vi "SPO2.vi"(5 "A":dbl=110.0 format="%#_13g", 7 "B":dbl=25.0 format="%#_13g", 8 "Inicial":u32, 9 "AMB":i16, 10 "IR":i16, 11 "RED":i16) -> (1 "Inicial Time Out":u32, 2 "Valor Medio":string, 3 "SpO2":string)   [LabVIEW 2013]
uses:
  <vilib>/Analysis/baseanly.llb/Mean (DBL).vi
  <vilib>/Analysis/NI_AALBase.lvlib
panel:
  out "Spo2 Array":dbl[](array[numeric])
  out "R":dbl
  out "VrmsIR":dbl
  out "VrmsRed":dbl
  out "VppIR":i16
  out "VppRed":i16
  out "MIN IR":dbl
  out "MIN IR":dbl
  out "MAX  IR":dbl
  out "MAX RED":dbl
  out "RED_ARRAY":i32[](array[numeric])
  out "IR_ARRAY":i32[](array[numeric])
  out "AMB_ARRAY":i32[](array[numeric])
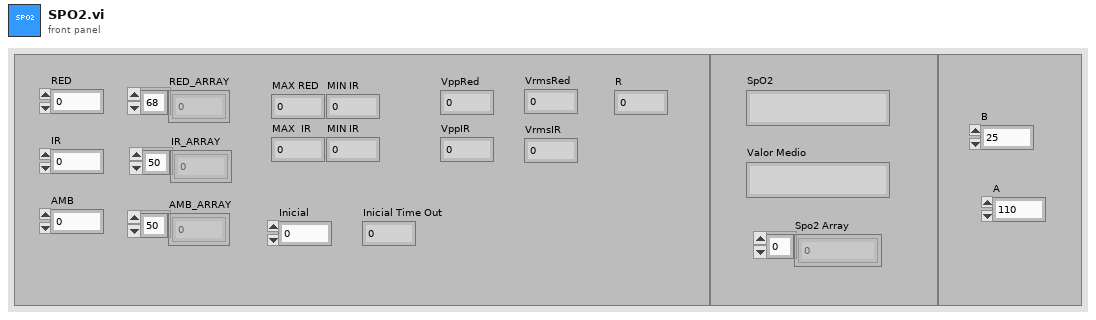
[diagram p1: front panel]
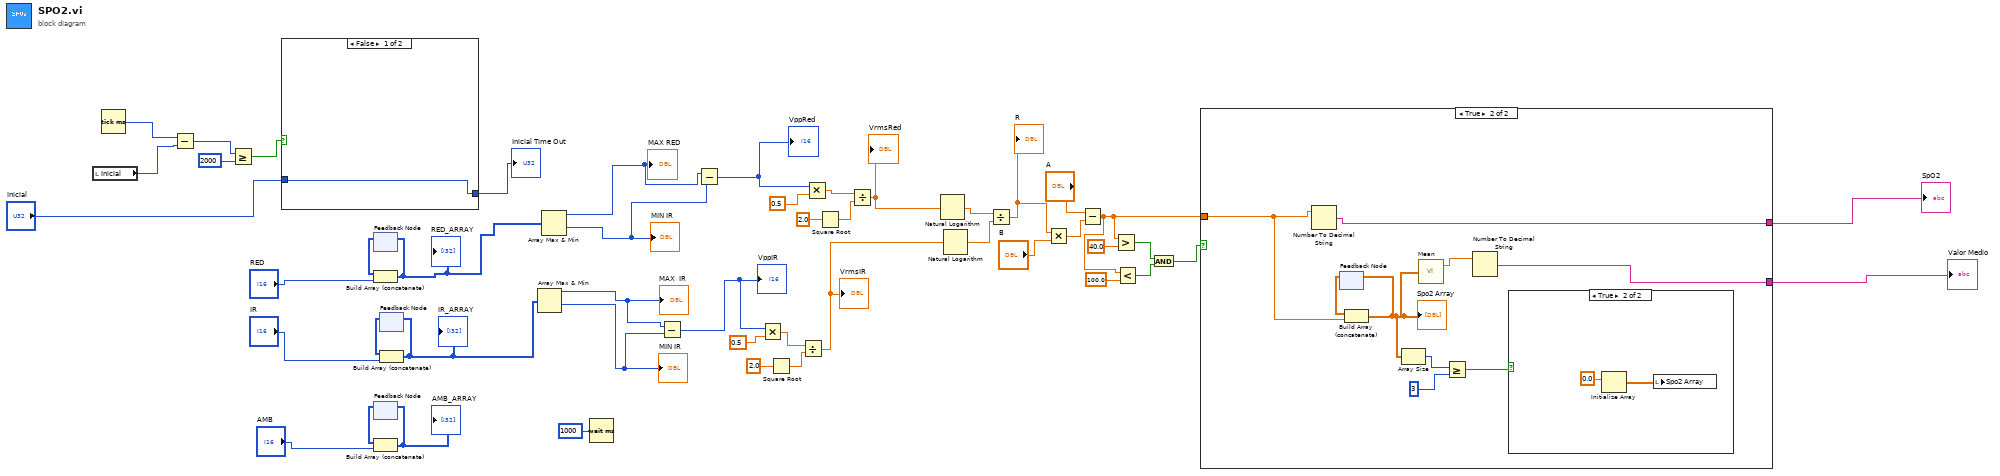
[diagram p0: block diagram]
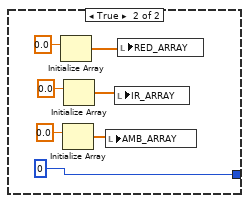
[diagram p2: hidden frame]
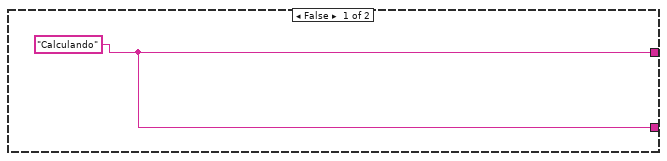
[diagram p3: hidden frame]
diagram:
  n1 = local read "Inicial"() -> (w3:u32)
  n2 = Tick Count (ms)() -> (millisecond timer value=w6:u32)
  n3 = Subtract(x=w6, y=w3) -> (x-y=w5:u32)
  n4 = Greater Or Equal?(x=w5, y=u32 2000) -> (x >= y?=w7:bool)
  n5 = case shown="False" w7 {
    tunnel: [w48 u32 0 ("Inicial Time")] -> w2
    tunnel: "Inicial" -> [w48 _]
    frame False {
    }
    frame True {
      n6 = Initialize Array(0.0 ("element")) -> (w52:dbl[])  [unwired: 1 in]
      n7 = Initialize Array(0.0 ("element")) -> (w50:dbl[])  [unwired: 1 in]
      n8 = Initialize Array(0.0 ("element")) -> (w51:dbl[])  [unwired: 1 in]
      n9 = local write "AMB_ARRAY"(w50) -> ()
      n10 = local write "IR_ARRAY"(w51) -> ()
      n11 = local write "RED_ARRAY"(w52) -> ()
    }
  }
  "Inicial Time Out" <- w2
  n12 = feedback #1() -> (w44:i16[])  [unwired: 1 in]
  n13 = Build Array (concatenate)(w44, "RED") -> (w43:i16[])
  "RED_ARRAY" <- w43
  n14 = feedback-in #1(w43) -> ()
  n15 = feedback #2() -> (w47:i16[])  [unwired: 1 in]
  n16 = Build Array (concatenate)(w47, "AMB") -> (w46:i16[])
  "AMB_ARRAY" <- w46
  n17 = feedback-in #2(w46) -> ()
  n18 = feedback #3() -> (w45:i16[])  [unwired: 1 in]
  n19 = Build Array (concatenate)(w45, "IR") -> (w39:i16[])
  "IR_ARRAY" <- w39
  n20 = feedback-in #3(w39) -> ()
  n21 = Array Max & Min(array=w39) -> (max value=w35:i16, min value=w34:i16)  [unwired: 2 out]
  "MAX  IR" <- w35
  "MIN IR" <- w34
  n22 = Array Max & Min(array=w43) -> (max value=w37:i16, min value=w36:i16)  [unwired: 2 out]
  "MAX RED" <- w37
  "MIN IR" <- w36
  n23 = Wait (ms)(milliseconds to wait=u32 1000) -> ()  [unwired: 1 out]
  n24 = Subtract(x=w35, y=w34) -> (x-y=w31:i16)
  "VppIR" <- w31
  n25 = Subtract(x=w37, y=w36) -> (x-y=w33:i16)
  "VppRed" <- w33
  n26 = Multiply(x=w31, y=0.5) -> (x*y=w29:dbl)
  n27 = Square Root(x=2.0) -> (sqrt(x)=w26:dbl)
  n28 = Divide(x=w29, y=w26) -> (x/y=w20:dbl)
  "VrmsIR" <- w20
  n29 = Multiply(x=w33, y=0.5) -> (x*y=w28:dbl)
  n30 = Square Root(x=2.0) -> (sqrt(x)=w27:dbl)
  n31 = Divide(x=w28, y=w27) -> (x/y=w21:dbl)
  "VrmsRed" <- w21
  n32 = Natural Logarithm(1:w21) -> (0:w22:dbl)
  n33 = Natural Logarithm(1:w20) -> (0:w23:dbl)
  n34 = Divide(x=w22, y=w23) -> (x/y=w19:dbl)
  "R" <- w19
  n35 = Multiply(x=w19, y="B") -> (x*y=w17:dbl)
  n36 = Subtract(x="A", y=w17) -> (x-y=w8:dbl)
  n37 = Greater?(x=w8, y=40.0) -> (0:w14:bool)
  n38 = Less?(x=w8, y=100.0) -> (x < y?=w15:bool)
  n39 = And(x=w14, y=w15) -> (x .and. y?=w13:bool)
  n40 = case shown="True" w13 {
    tunnel: [w56 w65] -> w10
    tunnel: w8 -> [_ w64]
    tunnel: [w56 w60] -> w9
    frame False {
      w56 = "Calculando" ("String")
    }
    frame True {
      n41 = Number To Decimal String(number=w64) -> (decimal integer string=w65:string)  [unwired: 1 in]
      n42 = feedback #4() -> (w63:dbl[])  [unwired: 1 in]
      n43 = Build Array (concatenate)(w63, w64) -> (w62:dbl[])
      "Spo2 Array" <- w62
      n44 = feedback-in #4(w62) -> ()
      n45 = Array Size(array=w62) -> (size(s)=w59:i32)
      n46 = call-poly <vilib>:"Mean.vi"("X"=w62) -> ("mean"=w61:dbl)  [unwired: 1 out]
      n47 = Greater Or Equal?(x=w59, y=3) -> (x >= y?=w58:bool)
      n48 = Number To Decimal String(number=w61) -> (decimal integer string=w60:string)  [unwired: 1 in]
      n49 = case shown="True" w58 {
        frame False {
        }
        frame True {
          n50 = Initialize Array(0.0 ("element")) -> (w67:dbl[])  [unwired: 1 in]
          n51 = local write "Spo2 Array"(w67) -> ()
        }
      }
    }
  }
  "SpO2" <- w10
  "Valor Medio" <- w9
